vi "McP Calibrate V1.00.vi"() -> ()   [LabVIEW 2025]
doc: "If you enter this program by mistake, click RETURN to quit.\n\nCALIBRATION STEPS:\n\n(0) Make sure you have calibration source (Ne lamp, Hg lamp, etc.) set up correctly.\n(1) Select a calibration line.\n(2) Click Calibrate.\n The spectrometer will move to the selected calibration line wavelength, take a CCD shot and fit the result.\n(3)Check the calibration result. You will be prompt whether to accept the result.\n (3a)Click \"Cancel\" to leave the system unaltered.\n (3b)If you click \"OK\", the counter position will be set to the calibrated value.\nThe spectrometer will return to the original internal (stepper) position afterward.\n\n\nAuthor: Scott Hannahs <sth@magnet.fsu.edu>\n\nThis software is licensed for use under the “MIT License\"\nCopyright (c) 2025 Scott Hannahs, sth@sth@magnet.sthnet.net\n\nPermission is hereby granted, free of charge, to any person obtaining a copy of this software and associated documentation files (the \"Software\"), to deal in the Software without restriction, including without limitation the rights to use, copy, modify, merge, publish, distribute, sublicense, and/or sell copies of the Software, and to permit persons to whom the Software is furnished to do so, subject to the following conditions: The above copyright notice and this permission notice shall be included in all copies or substantial portions of the Software.\n\nTHE SOFTWARE IS PROVIDED \"AS IS\", WITHOUT WARRANTY OF ANY KIND, EXPRESS OR IMPLIED, INCLUDING BUT NOT LIMITED TO THE WARRANTIES OF MERCHANTABILITY, FITNESS FOR A PARTICULAR PURPOSE AND NONINFRINGEMENT. IN NO EVENT SHALL THE AUTHORS OR COPYRIGHT HOLDERS BE LIABLE FOR ANY CLAIM, DAMAGES OR OTHER LIABILITY, WHETHER IN AN ACTION OF CONTRACT, TORT OR OTHERWISE, ARISING FROM, OUT OF OR IN CONNECTION WITH THE SOFTWARE OR THE USE OR OTHER DEALINGS IN THE SOFTWARE."
uses:
  Globals and TypeDefs/Global Varibal Control.vi
  Calibration/GlobalCalLampInfo.ctl
panel:
  in  "Return?":bool
  out "cursor position":dbl format="%.4f"
  in  "Points Between":i32=10 min=0 step=1
  out "Difference (cm-1)":dbl caption="(cm-1)" format="%.2e"
  out "Difference (meV)":dbl caption="(meV)" format="%.2e"
  out "Difference":dbl caption="(nm)" format="%.2e"
  out "Calibrated Wavelenth(nm)":dbl=1000.0 format="%.4f"
  out "peak plot (post-calibration)":cluster{"X-axis":dbl[], dbl[]}[](graph)
  out "Full plot":cluster{"X-axis":dbl[], "The Data":dbl[]}(graph)
  in  "Exposuretime (s)":dbl=0.5 format="%.2f"
  in  "CCD GPIB Address":u16=1
  out "Current WL":dbl=692.9467 caption="PreCalibrated Wavelength (nm)" format="%.4f"
  in  "Select WL":u16(ring)=6 caption="Select a Calibration Line" items=["808.2458  nm  ( Ne )", "794.3181  nm  ( Ne )", "743.8898  nm  ( Ne )", "724.5167  nm  ( Ne )", "717.3938  nm  ( Ne )", "703.2413  nm  ( Ne )", "692.9467  nm  ( Ne )", "671.7043  nm  ( Ne )", "667.8276  nm  ( Ne )", "659.8953  nm  ( Ne )", "653.2882  nm  ( Ne )", "650.6528  nm  ( Ne )", "640.2246  nm  ( Ne )", "638.2991  nm  ( Ne )", "633.4428  nm  ( Ne )", "632.8165  nm  ( Ne )", "579.2200  nm  ( Hg )", "577.1100  nm  ( Hg )", "546.2200  nm  ( Hg )", "435.9500  nm  ( Hg )", "407.8900  nm  ( Hg )", "404.7700  nm  ( Hg )", "366.4300  nm  ( Hg )", "365.5900  nm  ( Hg )", "365.1200  nm  ( Hg )", "Input Wavelength"]
  in  "StartCal":bool
  in  "Cal WL":dbl=692.9467 caption="Input Calibration Wavelength (nm)" format="%.4f"
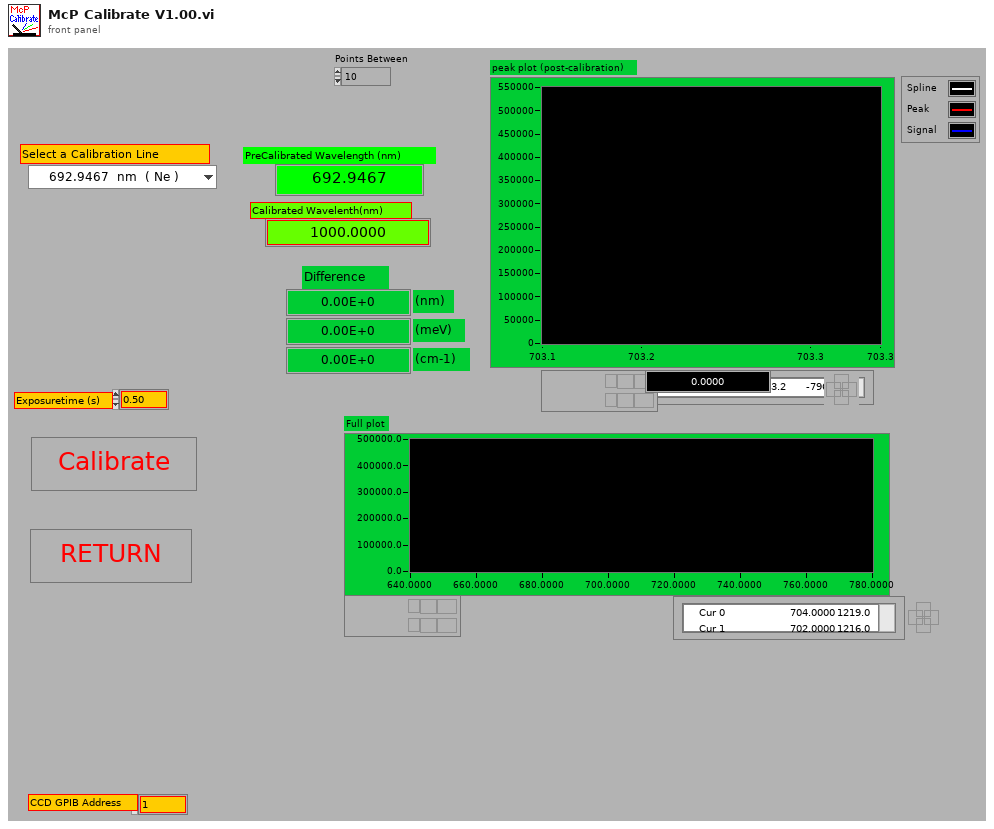
[diagram p1: front panel]
types:
  T1 = cluster{"Element":string, "Wavelength":dbl, "CalWidth":dbl}[]
  T2 = enum16{"Linear", "Polynomial", "Spline", "Rational"}
  T3 = cluster{"Element":string, "Wavelength":dbl, "CalWidth":dbl}
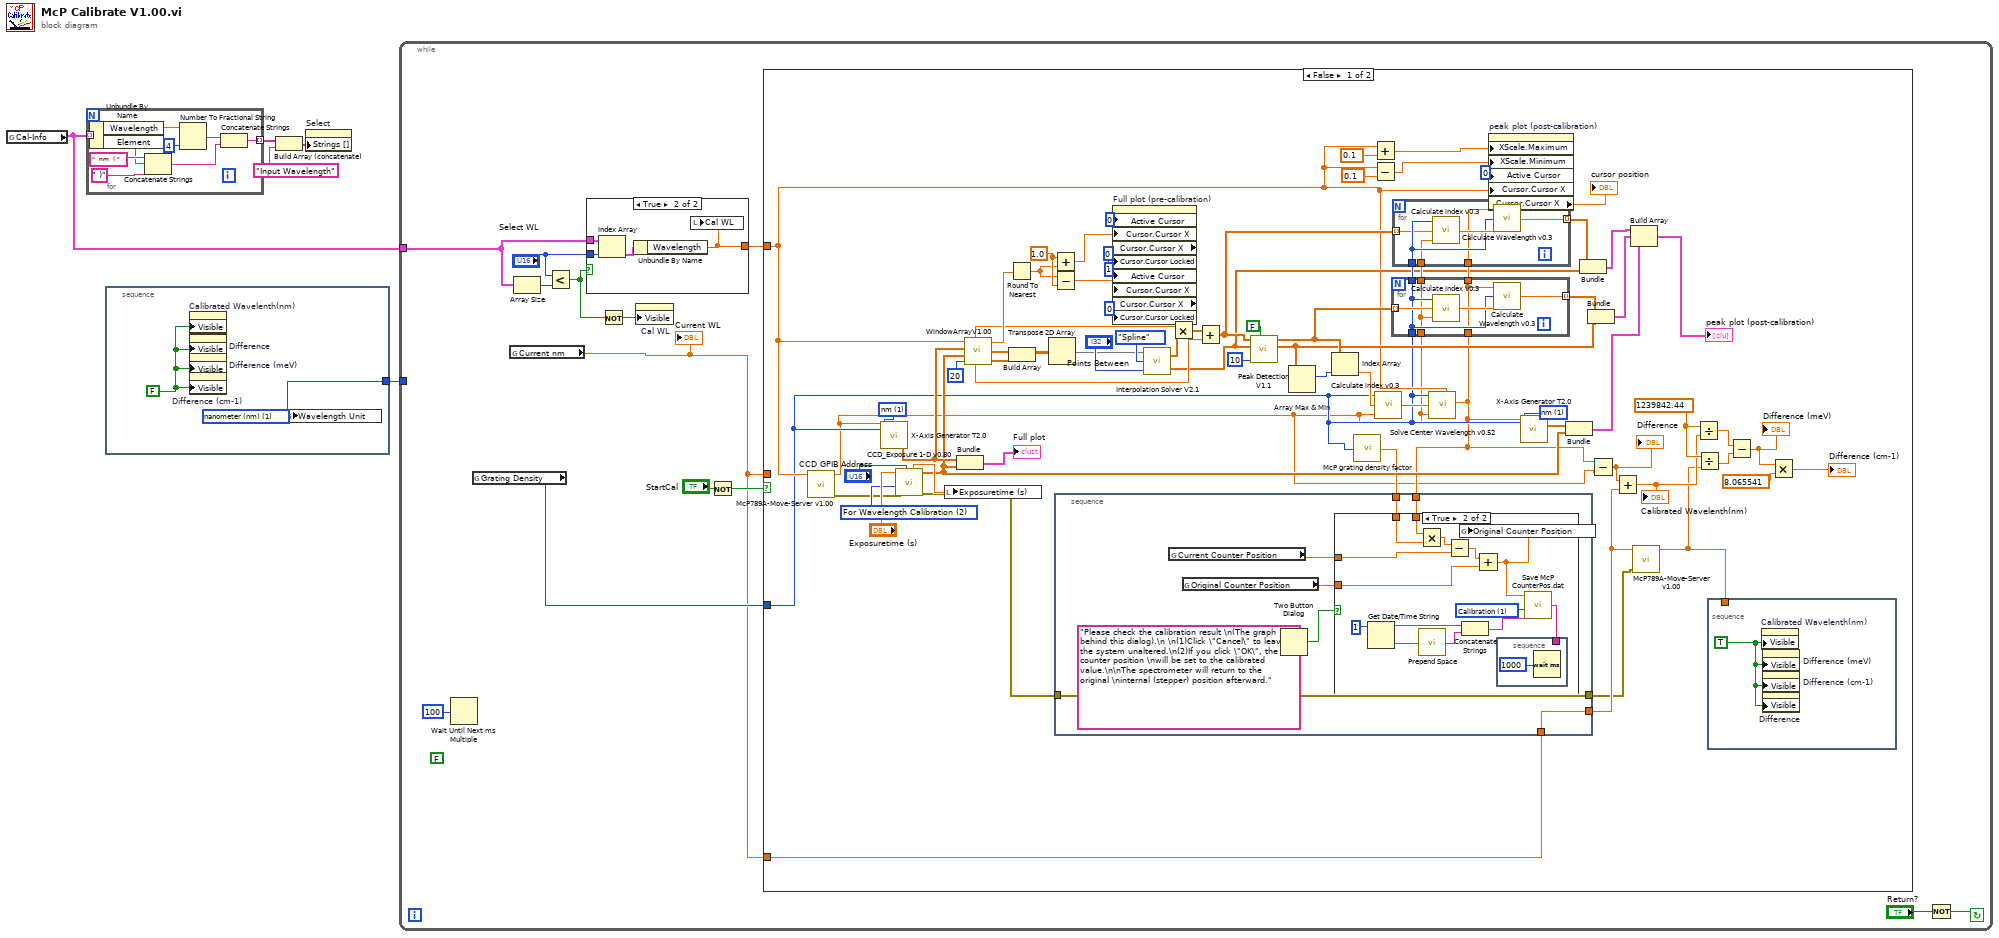
[diagram p0: block diagram]
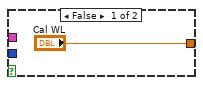
[diagram p2: hidden frame]
diagram:
  n1 = global read "GlobalCalLampInfo.ctl" "Cal-Info"() -> (w5:T1)
  n2 = for {
    tunnel: w5 -> [w14] mode=indexing
    tunnel: [w12] -> w4 mode=indexing
    n3 = Unbundle By Name(w14) -> ("Wavelength"=w11:dbl, "Element"=w8:string)
    n4 = Concatenate Strings("  nm  ( ", w8, " )") -> (w6:string)
    n5 = Number To Fractional String(number=w11, precision (6)=4) -> (F-format string=w10:string)  [unwired: 2 in]
    n6 = Concatenate Strings(w10, w6) -> (w12:string)
  }
  n7 = stacked-sequence {
    tunnel: [w15] -> w1
    frame #0 {
      w15 = u8 1 items=["Point #", "nanometer (nm)", "electron volt (eV)", "Milli eV (meV)", "Wavenumber (cm-1)"] ("Wavelength Unit")
      w16 = FALSE ("Visible")
      n8 = property on="Calibrated Wavelenth(nm)" class="DigNum (strict)"("Visible"=w16) -> ()  [unwired: 2 in, 2 out]
      n9 = property on="Difference" class="DigNum (strict)"("Visible"=w16) -> ()  [unwired: 2 in, 2 out]
      n10 = property on="Difference (meV)" class="DigNum (strict)"("Visible"=w16) -> ()  [unwired: 2 in, 2 out]
      n11 = property on="Difference (cm-1)" class="DigNum (strict)"("Visible"=w16) -> ()  [unwired: 2 in, 2 out]
      n12 = global write "Global Varibal Control.vi" "Wavelength Unit"(w15) -> ()
    }
  }
  n13 = Build Array (concatenate)(w4, "Input Wavelength") -> (w2:string[])
  n14 = property on="Select" class="Ring (strict)"("Strings []"=w2) -> ()  [unwired: 2 in, 2 out]
  n15 = while {
    tunnel: w1 -> [_]
    tunnel: w5 -> [w29]
    stop <- w19 continue-if-true
    (unwired) FALSE
    n16 = Wait Until Next ms Multiple(millisecond multiple=u32 100) -> ()  [unwired: 1 out]
    n17 = global read "Global Varibal Control.vi" "Grating Density"() -> (w18:u8)
    n18 = global read "Global Varibal Control.vi" "Current nm"() -> (w17:dbl)
    "Current WL" <- w17
    n19 = Array Size(array=w29) -> (size(s)=w25:i32)
    n20 = Less?(x="Select WL", y=w25) -> (x < y?=w22:bool)
    n21 = case shown="True" w22 {
      tunnel: ["Cal WL" w32] -> w28
      tunnel: w29 -> [_ w33]
      tunnel: "Select WL" -> [_ w31]
      frame False {
      }
      frame True {
        n22 = Index Array(array=w33, index=w31) -> (element=w34:T3)
        n23 = Unbundle By Name(w34) -> ("Wavelength"=w32:dbl)
        n24 = local write "Cal WL"(w32) -> ()
      }
    }
    n25 = Not(x=w22) -> (.not. x?=w23:bool)
    n26 = property on="Cal WL" class="DigNum (strict)"("Visible"=w23) -> ()  [unwired: 2 in, 2 out]
    n27 = Not(x="StartCal") -> (.not. x?=w21:bool)
    n28 = case shown="False" w21 {
      tunnel: w28 -> [w45 _]
      tunnel: w17 -> [w38 _]
      tunnel: w18 -> [w44 _]
      tunnel: w17 -> [_ _]
      frame False {
        w84 = 1 items=["Point #", "nm", "eV", "meV", "cm-1"] ("X-Axis Unit")
        w47 = 1239842.44
        w102 = 1.0
        w103 = 1 items=["Point #", "nm", "eV", "meV", "cm-1"] ("X-Axis Unit")
        w105 = u16 2 items=["No Over-Exposure Correction", "Over-Exposure Correction", "For Wavelength Calibration"] ("Mode")
        n29 = call "McP789A-Move-Server v1.00.vi"("GOTO"=w45) -> ("error out"=w104:errorcluster, "CurrentPosition"=w39:dbl)  [unwired: 7 in, 1 out]
        n30 = call "X-Axis Generator T2.0.vi"("Unit"=w44, "Grating Groove Density"=w103, "Central Wavelength"=w39) -> ("X-axis"=w94:dbl[])  [unwired: 3 out]
        n31 = call "CCD_Exposure 1-D v0.80.vi"("CCD GPIB Address"="CCD GPIB Address", "error in"=w104, "Mode"=w105, "Exposuretime (s)"="Exposuretime (s)") -> ("Error Out"=w36:errorcluster, "The Data"=w82:dbl[], "Exposuretime (s) out"=w89:dbl)  [unwired: 1 in, 4 out]
        n32 = local write "Exposuretime (s)"(w89) -> ()
        n33 = Bundle("X-axis"=w94, "The Data"=w82) -> (→"Full plot":cluster{"X-axis":dbl[], "The Data":dbl[]})  [unwired: 1 in]
        n34 = call "WindowArrayV1.00.vi"("Searching center"=w45, "X-axis"=w94, "The Data"=w82, "Window Width (point)"=20) -> ("scale"=w80:dbl, "starting point"=w79:dbl, "Closest peak position"=w93:dbl, "X-Axis Subset"=w66:dbl[], "Data Subset"=w65:dbl[])
        n35 = Round To Nearest(number=w93) -> (nearest integer value=w101:dbl)
        n36 = Build Array(w66, w65) -> (w68:dbl[][])
        n37 = Transpose 2D Array(2D array=w68) -> (transposed array=w67:dbl[][])
        n38 = Add(x=w102, y=w101) -> (x+y=w96:dbl)
        n39 = Subtract(x=w101, y=w102) -> (x-y=w95:dbl)
        n40 = property on="Full plot (pre-calibration)" class="XYGraph (strict)" props=["Active Cursor", "Cursor", "Cursor X", "Cursor", "Cursor X", "Cursor", "Cursor Locked", "Active Cursor", "Cursor", "Cursor X", "Cursor", "Cursor X", "Cursor", "Cursor Locked"]("Active Cursor"=u32 0, "Cursor.Cursor X"=w96, "Cursor.Cursor Locked"=u32 0 ("Cursor Locked"), "Active Cursor"=u32 1, "Cursor.Cursor X"=w95, "Cursor.Cursor Locked"=u32 0 ("Cursor Locked")) -> ()  [unwired: 2 in, 4 out]
        n41 = call "Interpolation Solver V2.1.vi"("Points Between"="Points Between", "Type of Interpolation"=T2."Spline", "Data"=w67) -> ("Interpolated Data"=w53:dbl[], "Interpolated X Axis"=w64:dbl[])
        n42 = Multiply(x=w80, y=w64) -> (x*y=w78:dbl[])
        n43 = Add(x=w78, y=w79) -> (x+y=w55:dbl[])
        n44 = call "Peak Detection V1.1.vi"("View Result?"=FALSE, "PD width"=10 ("Points Between"), "Input y data"=w53, "Input x data"=w55) -> ("Peak Amplitudes"=w52:dbl[], "Peak Locations"=w59:dbl[])  [unwired: 1 in, 5 out]
        n45 = Array Max & Min(array=w52) -> (max index (indices)=w77:i32)  [unwired: 3 out]
        n46 = Index Array(array=w59, index=w77) -> (element=w76:dbl)
        n47 = call "McP grating density factor.vi"("Grating Density"=w44) -> ("GratingFactor"=w46:dbl)
        n48 = Add(x=w45, y=0.1) -> (x+y=w72:dbl)
        n49 = Subtract(x=w45, y=0.1) -> (x-y=w71:dbl)
        n50 = call "Calculate index v0.3.vi"("Central Wavelength"=w39, "Current Wavelength"=w76, "Current Grating Density"=w44) -> ("index (out)"=w60:dbl)  [unwired: 2 in]
        n51 = call "Solve Center Wavelength v0.52.vi"("Standard Wavelength"=w45, "Current Central Wavelength"=w39, "pixel index"=w60, "Current Grating Density"=w44) -> ("Calibrated Central Wavelength"=w43:dbl)  [unwired: 4 in]
        n52 = stacked-sequence {
          tunnel: w46 -> [w115]
          tunnel: w43 -> [w114]
          tunnel: [w109] -> w37
          tunnel: w38 -> [w109]
          tunnel: w36 -> [w108]
          tunnel: [w108] -> w35
          frame #0 {
            n53 = global read "Global Varibal Control.vi" "Current Counter Position"() -> (w111:dbl)
            n54 = global read "Global Varibal Control.vi" "Original Counter Position"() -> (w110:dbl)
            n55 = Two Button Dialog(message="Please check the calibration result \n(The graph behind this dialog).\n \n(1)Click \"Cancel\" to leave the system unaltered.\n(2)If you click \"OK\", the counter position \nwill be set to the calibrated value.\n\nThe spectrometer will return to the original \ninternal (stepper) position afterward.") -> (T button?=w113:bool)  [unwired: 2 in]
            n56 = case shown="True" w113 {
              tunnel: w111 -> [_ w129]
              tunnel: w115 -> [_ w122]
              tunnel: w114 -> [_ w121]
              tunnel: w110 -> [_ w118]
              frame False {
              }
              frame True {
                w128 = u16 1 items=["Moving", "Calibration", "Key in", "Initialization"] ("Set Method")
                n57 = Get Date/Time String(date format (0)=1) -> (date string=w124:string, time string=w126:string)  [unwired: 2 in]
                n58 = Multiply(x=w121, y=w122) -> (x*y=w120:dbl)
                n59 = call "Prepend Space.vi"("Input String"=w126) -> ("Space + Input String"=w125:string)
                n60 = Subtract(x=w120, y=w129) -> (x-y=w119:dbl)
                n61 = Concatenate Strings(w124, w125) -> (w123:string)
                n62 = Add(x=w119, y=w118) -> (x+y=w117:dbl)
                n63 = global write "Global Varibal Control.vi" "Original Counter Position"(w117) -> ()
                n64 = call "Save McP CounterPos.dat.vi"("Last Calibration Date"=w123, "Set Method"=w128, "McP Counter Position"=w117) -> ("Written content"=w116:string)  [unwired: 3 in]
                n65 = stacked-sequence {
                  tunnel: w116 -> [_]
                  frame #0 {
                    n66 = Wait (ms)(milliseconds to wait=u32 1000) -> ()  [unwired: 1 out]
                  }
                }
              }
            }
          }
        }
        n67 = for {
          tunnel: w43 -> [w139]
          tunnel: w39 -> [w140]
          tunnel: w44 -> [w141]
          tunnel: w59 -> [w142] mode=indexing
          tunnel: [w141] -> w58
          tunnel: [w140] -> w56
          tunnel: [w139] -> w57
          tunnel: [w138] -> w51 mode=indexing
          n68 = call "Calculate index v0.3.vi"("Central Wavelength"=w140, "Current Wavelength"=w142, "Current Grating Density"=w141) -> ("index (out)"=w143:dbl)  [unwired: 2 in]
          n69 = call "Calculate Wavelength v0.3.vi"("pixel index"=w143, "Current Grating Density"=w141, "Central Wavelength"=w139) -> ("nm (out)"=w138:dbl)  [unwired: 2 in]
        }
        n70 = for {
          tunnel: w57 -> [w135]
          tunnel: w58 -> [w136]
          tunnel: w55 -> [w134] mode=indexing
          tunnel: w56 -> [w133]
          tunnel: [w132] -> w54 mode=indexing
          n71 = call "Calculate index v0.3.vi"("Central Wavelength"=w133, "Current Wavelength"=w134, "Current Grating Density"=w136) -> ("index (out)"=w137:dbl)  [unwired: 2 in]
          n72 = call "Calculate Wavelength v0.3.vi"("pixel index"=w137, "Current Grating Density"=w136, "Central Wavelength"=w135) -> ("nm (out)"=w132:dbl)  [unwired: 2 in]
        }
        n73 = property on="peak plot (post-calibration)" class="XYGraph (strict)"("XScale.Maximum"=w72, "XScale.Minimum"=w71, "Active Cursor"=u32 0, "Cursor.Cursor X"=w45) -> ("Cursor.Cursor X"=→"cursor position":dbl)  [unwired: 2 in, 2 out]
        n74 = call "X-Axis Generator T2.0.vi"("Unit"=w44, "Grating Groove Density"=w84, "Central Wavelength"=w43) -> ("X-axis"=w83:dbl[])  [unwired: 3 out]
        n75 = Bundle("X-axis"=w83, "The Data"=w82) -> (w75:cluster{"X-axis":dbl[], "The Data":dbl[]})  [unwired: 1 in]
        n76 = Bundle(w54, "Interpolated Data"=w53) -> (w63:cluster{dbl[], "Interpolated Data":dbl[]})  [unwired: 1 in]
        n77 = Bundle(w51, "Peak Amplitudes"=w52) -> (w62:cluster{dbl[], "Peak Amplitudes":dbl[]})  [unwired: 1 in]
        n78 = Subtract(x=w43, y=w39) -> (x-y=w40:dbl)
        "Difference" <- w40
        n79 = Add(x=w40, y=w37) -> (x+y=w42:dbl)
        "Calibrated Wavelenth(nm)" <- w42
        n80 = Build Array(w63, w62, w75) -> (→"peak plot (post-calibration)":cluster{"X-axis":dbl[], "The Data":dbl[]}[])
        n81 = call "McP789A-Move-Server v1.00.vi"("error in"=w35, "GOTO"=w37) -> ("CurrentPosition"=w41:dbl)  [unwired: 6 in, 2 out]
        n82 = Divide(x=w47, y=w42) -> (x/y=w88:dbl)
        n83 = Divide(x=w47, y=w41) -> (x/y=w87:dbl)
        n84 = stacked-sequence {
          tunnel: w41 -> [_]
          frame #0 {
            w131 = TRUE
            n85 = property on="Calibrated Wavelenth(nm)" class="DigNum (strict)"("Visible"=w131) -> ()  [unwired: 2 in, 2 out]
            n86 = property on="Difference (meV)" class="DigNum (strict)"("Visible"=w131) -> ()  [unwired: 2 in, 2 out]
            n87 = property on="Difference (cm-1)" class="DigNum (strict)"("Visible"=w131) -> ()  [unwired: 2 in, 2 out]
            n88 = property on="Difference" class="DigNum (strict)"("Visible"=w131) -> ()  [unwired: 2 in, 2 out]
          }
        }
        n89 = Subtract(x=w88, y=w87) -> (x-y=w86:dbl)
        "Difference (meV)" <- w86
        n90 = Multiply(x=w86, y=8.065541) -> (x*y=→"Difference (cm-1)":dbl)
      }
      frame True {
      }
    }
    n91 = Not(x="Return?") -> (.not. x?=w19:bool)
  }
